vi "Reset Metodo.vi"(8 "error in (no error)":errorcluster, 11 "TektroniksTDS in":refnum<class "TektroniksTDS.lvclass">) -> (0 "error out":errorcluster, 3 "TektroniksTDS out":refnum<class "TektroniksTDS.lvclass">)   [LabVIEW 2020, in "TektroniksTDS.lvclass"]
uses:
  TektroniksTDS.lvclass
  Osciloscope/Osciloscope.lvclass
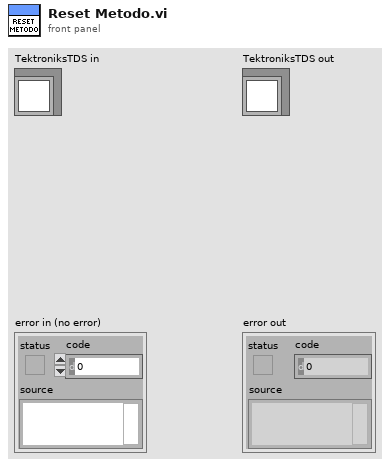
[diagram p1: front panel]
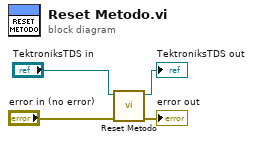
[diagram p0: block diagram]
diagram:
  n1 = call-parent "Reset Metodo.vi"("error in (no error)"="error in (no error)", "Osciloscope in"="TektroniksTDS in") -> ("error out"=→"error out":errorcluster, "Osciloscope out"=→"TektroniksTDS out":refnum<class "TektroniksTDS.lvclass">)  [unwired: 8 in]
